vi "SL Source.vi"(8 "error in (no error)":errorcluster, 10 "settling time (s)":dbl format="%#_6p", 11 "voltage level (V)":dbl) -> (0 "error out":errorcluster)   [LabVIEW 2019]
uses:
  Globals.vi
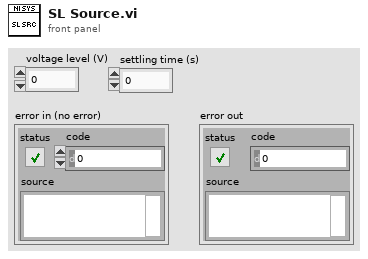
[diagram p1: front panel]
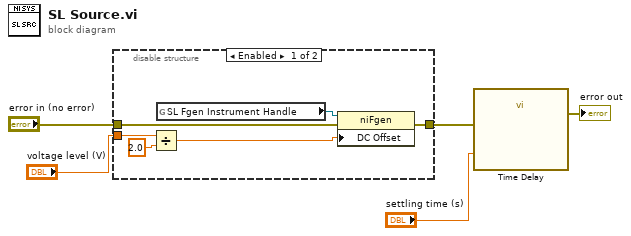
[diagram p0: block diagram]
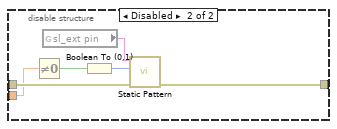
[diagram p2: hidden frame]
diagram:
  n1 = disable-structure shown="Enabled" {
    disable-tunnel: "voltage level (V)" -> [w8 w13]
    disable-tunnel: "error in (no error)" -> [w7 w14]
    disable-tunnel: [w6 w12] -> w2
    frame Enabled {
      n2 = Divide(x=w8, y=2.0) -> (x/y=w9:dbl)
      n3 = global read "Globals.vi" "SL Fgen Instrument Handle"() -> (w11:refnum<k15>)
      n4 = property class="niFgen"(reference=w11, error in=w7, "DC Offset"=w9) -> (error out=w6:errorcluster)  [unwired: 1 out]
    }
    frame Disabled {
      n5 = Not Equal To 0?(x=w13) -> (x != 0?=w15:bool)
      n6 = global read "Globals.vi" "sl_ext pin"() -> (w17:string)
      n7 = Boolean To (0,1)(Boolean=w15) -> (0, 1=w16:i16)
      n8 = call "Static Pattern.vi"("error in (no error)"=w14, "write data (0x0000)"=w16, "channel list (all:\"\")"=w17) -> ("error out"=w12:errorcluster)  [unwired: 8 in]
    }
  }
  n9 = call "Time Delay"("error in (no error)"=w2, "Delay Time (s)"="settling time (s)") -> ("error out"=→"error out":errorcluster)  [unwired: 9 in]
